vi "testing_test1.vi"() -> ()   [LabVIEW 2015]
uses:
  <vilib>/LabVIEW Interface for Arduino/LabVIEW Interface for Arduino.lvlib
panel:
  out "Tab Control":T1
  out "?":string
  in  "Exit the program":bool
  in  "Start Test":bool
  in  "Next Button 2":bool
  out "String 2":string
  in  "Next Button 3":bool
  out "String 3":string
  in  "stop 3":bool
  in  "Next Button 4":bool
  out "String 4":string
  in  "stop K1":bool
  out "Error K1":string
  out "Error K2":string
  in  "stop 2":bool
  in  "Complete K2":bool
  out "Last  Message 2":string
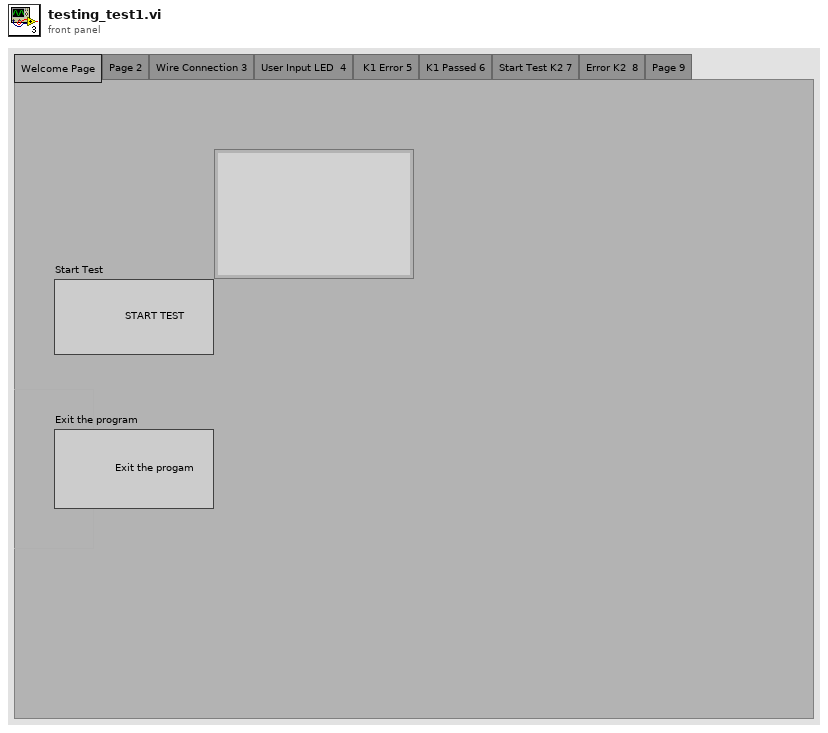
[diagram p1: front panel]
types:
  T1 = typedef "Control 1" = enum32{"Welcome Page", "Page 2", "Wire Connection 3", "User Input LED  4", " K1 Error 5", "K1 Passed 6", "Start Test K2 7", "Error K2  8", "Page 9"}
  T2 = enum32{"Page 1", "Page 2", "Page 3", "Page 4", "Page 5", "Page 6", "Page 7", "Page 8", "Page 9"}
  T3 = enum32{"Welcome Page 1", "Page 2", "Wire Connection 3", "User Input LED 4", "K1 Error 5", "K1 Passed 6", "Start Test K2 7", "Error K2 8", "Page 9"}
  T4 = typedef "LabVIEW Interface for Arduino.lvlib/Arduino Resource.ctl" = cluster{"VISA resource":refnum<visa-resource-name>, "Board Type":T5, "Connection Type":enum8{"USB / Serial"}, "Bytes Per Packet (15)":u8}
  T5 = typedef "LabVIEW Interface for Arduino.lvlib/Board Type.ctl" = enum16{"Uno", "Dimuelanove w/Atmega 328", "Mega 2560"}
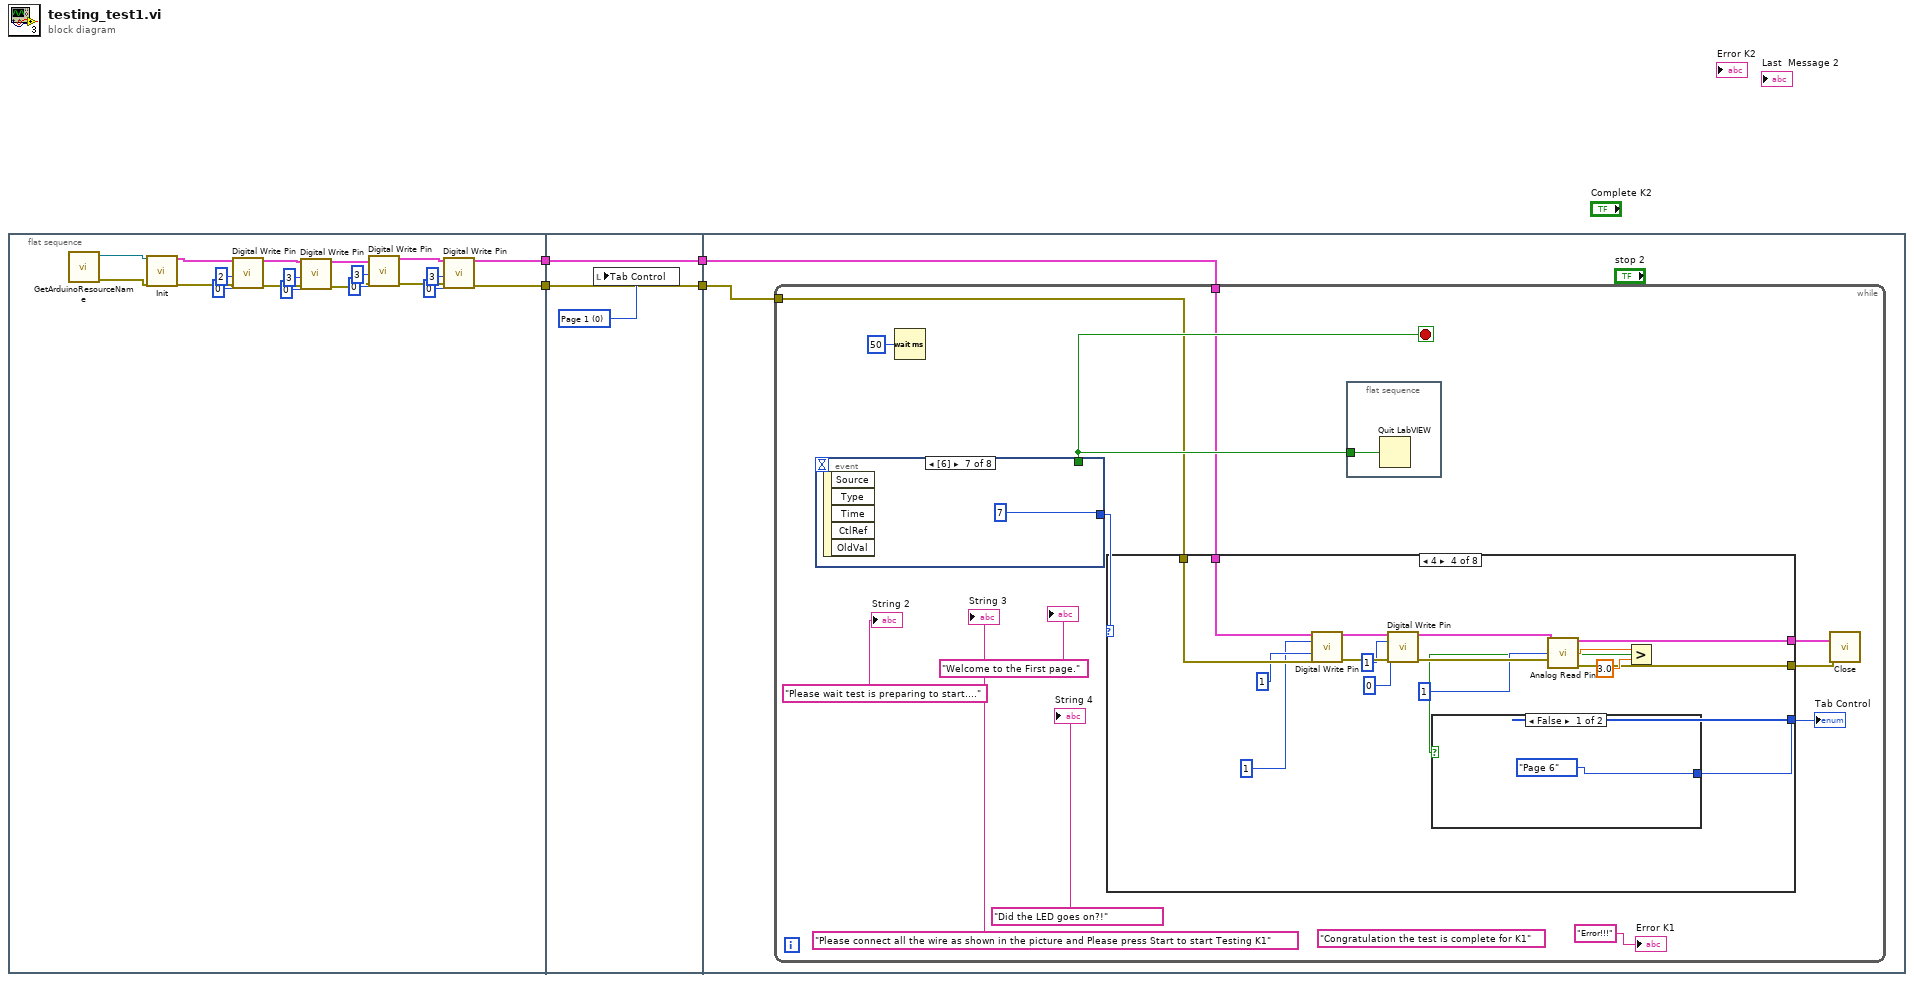
[diagram p0: block diagram]
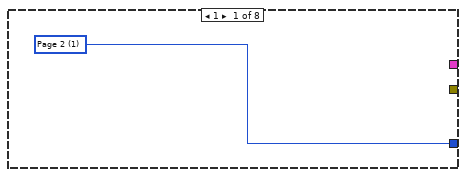
[diagram p2: hidden frame]
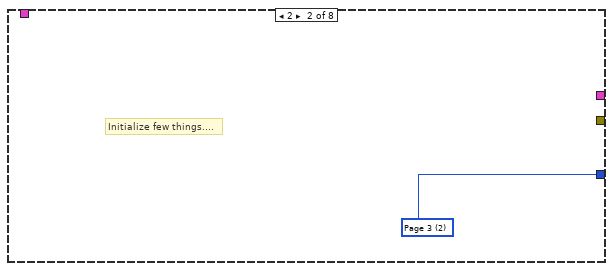
[diagram p3: hidden frame]
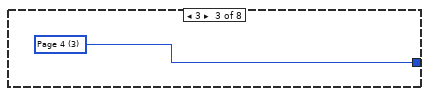
[diagram p4: hidden frame]
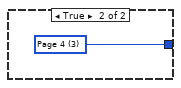
[diagram p5: hidden frame]
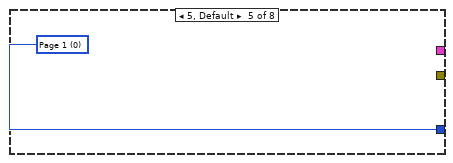
[diagram p6: hidden frame]
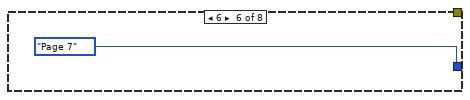
[diagram p7: hidden frame]
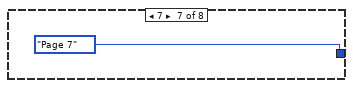
[diagram p8: hidden frame]
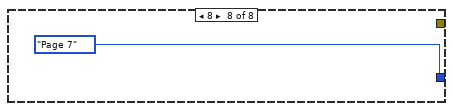
[diagram p9: hidden frame]
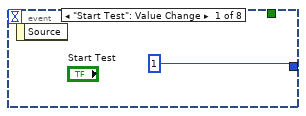
[diagram p10: hidden frame]
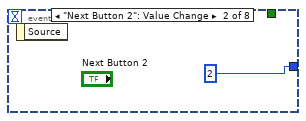
[diagram p11: hidden frame]
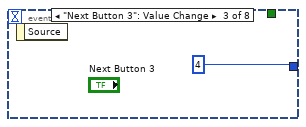
[diagram p12: hidden frame]
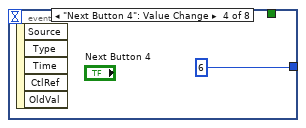
[diagram p13: hidden frame]
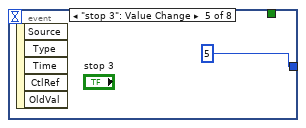
[diagram p14: hidden frame]
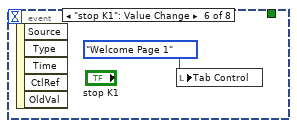
[diagram p15: hidden frame]
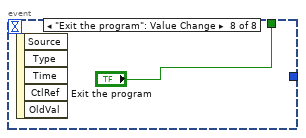
[diagram p16: hidden frame]
diagram:
  n1 = flat-sequence {
    tunnel: [w6] -> w3
    tunnel: [w5] -> w1
    tunnel: [w26] -> w4
    tunnel: w3 -> [w26]
    tunnel: [w25] -> w2
    tunnel: w1 -> [w25]
    tunnel: w4 -> [w29]
    tunnel: w2 -> [w28]
    frame #0 {
      n2 = call "GetArduinoResourceName.vi"() -> ("error out"=w19:errorcluster, "VISA resource name"=w20:refnum<visa-resource-name>)  [unwired: 10 in]
      n3 = call <vilib>:"Init.vi"("VISA resource"=w20, "error in"=w19) -> ("Arduino Resource"=w24:T4, "error out"=w23:errorcluster)  [unwired: 16 in]
      n4 = call <vilib>:"Digital Write Pin.vi"("Arduino Resource"=w24, "Digital I/O Pin (0)"=u8 2 ("Digital I/O Pin"), "Value (0)"=u8 0, "error in"=w23) -> ("Arduino Resource"=w12:T4, "error out"=w11:errorcluster)  [unwired: 10 in]
      n5 = call <vilib>:"Digital Write Pin.vi"("Arduino Resource"=w12, "Digital I/O Pin (0)"=u8 3 ("Digital I/O Pin"), "Value (0)"=u8 0, "error in"=w11) -> ("Arduino Resource"=w10:T4, "error out"=w9:errorcluster)  [unwired: 10 in]
      n6 = call <vilib>:"Digital Write Pin.vi"("Arduino Resource"=w10, "Digital I/O Pin (0)"=u8 3 ("Digital I/O Pin"), "Value (0)"=u8 0, "error in"=w9) -> ("Arduino Resource"=w8:T4, "error out"=w7:errorcluster)  [unwired: 10 in]
      n7 = call <vilib>:"Digital Write Pin.vi"("Arduino Resource"=w8, "Digital I/O Pin (0)"=u8 3 ("Digital I/O Pin"), "Value (0)"=u8 0, "error in"=w7) -> ("Arduino Resource"=w6:T4, "error out"=w5:errorcluster)  [unwired: 10 in]
    }
    frame #1 {
      w27 = u16 0 items=["Page 1"]
      n8 = local write "Tab Control"(w27) -> ()
    }
    frame #2 {
      n9 = while {
        tunnel: w29 -> [w34]
        tunnel: w28 -> [w33]
        stop <- w38 stop-if-true
        w35 = "Congratulation the test is complete for K1" ("Last  Message")
        n10 = event shown="[6]" {
          selector: _ -> [_ _ _ _ _ _ _ _]
          dyn-events: _ -> [_ _ _ _ _ _ _ _]
          timeout: _ -> [_ _ _ _ _ _ _ _]
          tunnel: [1 2 4 6 5 _ 7 _] -> w42
          tunnel: [_ _ _ _ _ _ _ "Exit the program"] -> w38
          event "Start Test": Value Change {
            n11 = event-data() -> ()  [unwired: 1 in, 1 out]
          }
          event "Next Button 2": Value Change {
            n12 = event-data() -> ()  [unwired: 1 in, 1 out]
          }
          event "Next Button 3": Value Change {
            n13 = event-data() -> ()  [unwired: 1 in, 1 out]
          }
          event "Next Button 4": Value Change {
            n14 = event-data() -> ()  [unwired: 1 in, 5 out]
          }
          event "stop 3": Value Change {
            n15 = event-data() -> ()  [unwired: 1 in, 5 out]
          }
          event "stop K1": Value Change {
            n16 = event-data() -> ()  [unwired: 1 in, 5 out]
            n17 = local write "Tab Control"(T3."Welcome Page 1" ("Tab Control")) -> ()
          }
          event #6 (no event record) {
            n18 = event-data() -> ()  [unwired: 1 in, 5 out]
          }
          event "Exit the program": Value Change {
            n19 = event-data() -> ()  [unwired: 1 in, 5 out]
          }
        }
        n20 = Wait (ms)(milliseconds to wait=u32 50) -> ()  [unwired: 1 out]
        n21 = case shown="4" w42 {
          tunnel: [w44 w45 w46 w52 w66 T2."Page 7" ("Tab Control") T2."Page 7" ("Tab Control") T2."Page 7" ("Tab Control")] -> w36
          tunnel: w34 -> [_ _ _ w63 _ _ _ _]
          tunnel: w33 -> [_ _ _ w62 _ _ _ _]
          tunnel: [_ _ _ w48 _ _ _ _] -> w31
          tunnel: [_ _ _ w47 _ _ _ _] -> w30
          frame 1 {
            w44 = u16 1 items=["Page 1", "Page 2", "Page 3"]
          }
          frame 2 {
            w45 = u16 2 items=["Page 1", "Page 2", "Page 3", "Page 4"]
            # "Initialize few things...."
          }
          frame 3 {
            w46 = u16 3 items=["Page 1", "Page 2", "Page 3", "Page 4", "Page 5"]
          }
          frame 4 {
            n22 = call <vilib>:"Digital Write Pin.vi"("Arduino Resource"=w63, "Digital I/O Pin (0)"=u8 1, "Value (0)"=u8 1 ("Digital I/O Pin (0)"), "error in"=w62) -> ("Arduino Resource"=w60:T4, "error out"=w59:errorcluster)  [unwired: 10 in]
            n23 = call <vilib>:"Digital Write Pin.vi"("Arduino Resource"=w60, "Digital I/O Pin (0)"=u8 1 ("Digital I/O Pin"), "Value (0)"=u8 0, "error in"=w59) -> ("Arduino Resource"=w56:T4, "error out"=w55:errorcluster)  [unwired: 10 in]
            n24 = call <vilib>:"Analog Read Pin.vi"("Arduino Resource"=w56, "Analog Input Pin (0)"=u8 1, "error in"=w55) -> ("Arduino Resource"=w48:T4, "Voltage"=w51:dbl, "error out"=w47:errorcluster)  [unwired: 10 in]
            n25 = Greater?(x=w51, y=3.0) -> (0:w50:bool)
            n26 = case shown="False" w50 {
              tunnel: [T2."Page 6" ("Tab Control") w65] -> w52
              frame False {
              }
              frame True {
                w65 = u16 3 items=["Page 1", "Page 2", "Page 3", "Page 4", "Page 5"]
              }
            }
          }
          frame 5, Default {
            w66 = u16 0 items=["Page 1"]
          }
          frame 6 {
          }
          frame 7 {
          }
          frame 8 {
          }
        }
        "Tab Control" <- w36
        n27 = flat-sequence {
          tunnel: w38 -> [w78]
          frame #0 {
            n28 = Quit LabVIEW(quit? (T)=w78) -> ()
          }
        }
        n29 = call <vilib>:"Close.vi"("Arduino Resource"=w31, "error in"=w30) -> ()  [unwired: 13 in, 1 out]
        "?" <- "Welcome to the First page."
        "String 2" <- "Please wait test is preparing to start...."
        "String 3" <- "Please connect all the wire as shown in the picture and Please press Start to start Testing K1"
        "String 4" <- "Did the LED goes on?!"
        "Error K1" <- "Error!!!" ("Error")
      }
    }
  }
